vi "Set Resistance Colors.vi"(8 "error in (no error)":errorcluster, 11 "Data in":T1 {"#Bands" min=3 max=6 step=1}) -> (0 "error out":errorcluster, 3 "Data out":T1 {"#Bands" min=3 max=6 step=1})   [LabVIEW 2018]
uses:
  Data--cluster.ctl
  Digit--enum.ctl
  Multiplier--enum.ctl
  Tolerance--enum.ctl
  Temp Coeficient--enum.ctl
  E-Series Reader/Series Data--cluster.ctl
  In Low Series--cluster.ctl
  In Mid-High Series--cluster.ctl
  Number of Bands--number.ctl
  Enum to Color Converters/Enum to Color Converters.lvlib
  E-Series Reader/E-Series Reader.lvlib
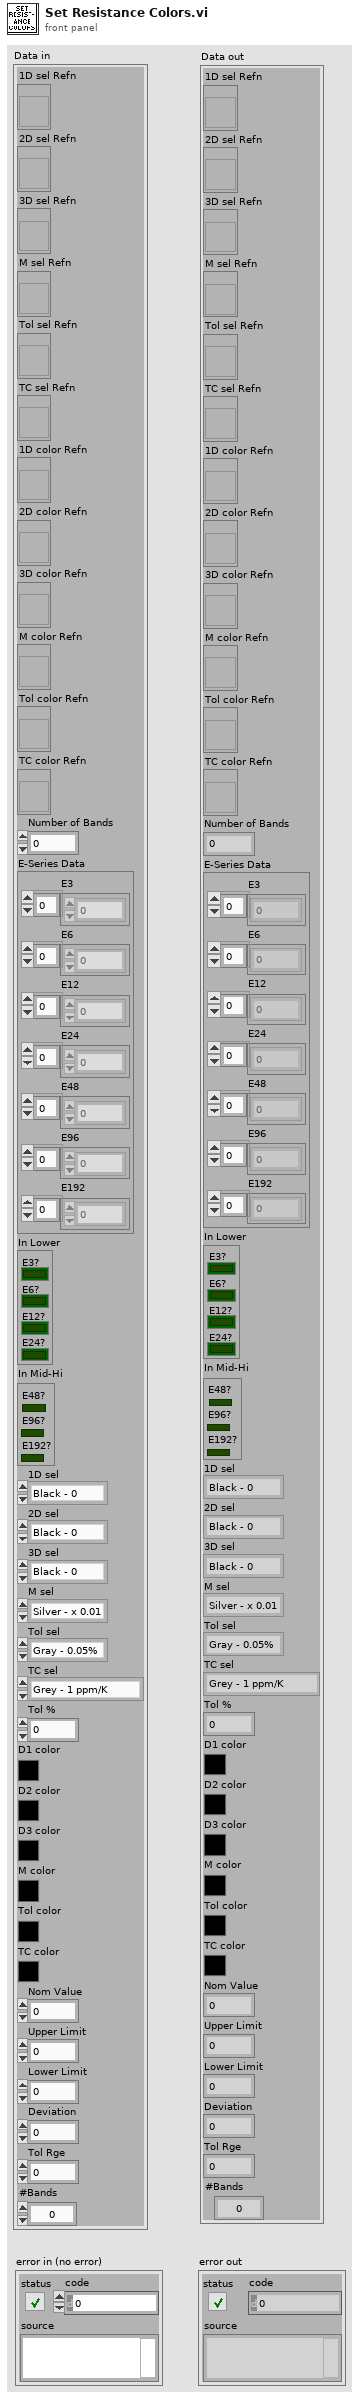
[diagram p1: front panel]
types:
  T1 = typedef "Data--cluster.ctl" = cluster{"1D sel Refn":refnum<vi>, "2D sel Refn":refnum<vi>, "3D sel Refn":refnum<vi>, "M sel Refn":refnum<vi>, "Tol sel Refn":refnum<vi>, "TC sel Refn":refnum<vi>, "1D color Refn":refnum<vi>, "2D color Refn":refnum<vi>, "3D color Refn":refnum<vi>, "M color Refn":refnum<vi>, "Tol color Refn":refnum<vi>, "TC color Refn":refnum<vi>, "Number of Bands":u8, "E-Series Data":T2, "In Lower":T3, "In Mid-Hi":T4, "1D sel":T5, "2D sel":T5, "3D sel":T5, "M sel":T6, "Tol sel":T7, "TC sel":T8, "Tol %":dbl, "D1 color":u32, "D2 color":u32, "D3 color":u32, "M color":u32, "Tol color":u32, "TC color":u32, "Nom Value":dbl, "Upper Limit":dbl, "Lower Limit":dbl, "Deviation":dbl, "Tol Rge":dbl, "#Bands":T9}
  T2 = typedef "E-Series Reader.lvlib/series data--cluster.ctl" = cluster{"E3":u16[], "E6":u16[], "E12":u16[], "E24":u16[], "E48":u16[], "E96":u16[], "E192":u16[]}
  T3 = typedef "In low series--cluster.ctl" = cluster{"E3?":bool, "E6?":bool, "E12?":bool, "E24?":bool}
  T4 = typedef "In mid-high series--cluster.ctl" = cluster{"E48?":bool, "E96?":bool, "E192?":bool}
  T5 = typedef "digit--enum.ctl" = enum16{"Black - 0", "Brown - 1", "Red - 2", "Orange - 3", "Yellow - 4", "Green - 5", "Blue - 6", "Violet - 7", "Grey - 8", "White - 9"}
  T6 = typedef "multiplier--enum.ctl" = enum16{"Silver - x 0.01", "Gold - x 0.1 ", "Black - x 1", "Brown - x 10", "Red - x 100", "Orange - x 1k", "Yellow - x 10k", "Green - 100k", "Blue - x 1M", "Violet - x10 M", "Grey - x 100M", "White - x 1G"}
  T7 = typedef "tolerance--enum.ctl" = enum16{"Gray - 0.05%", "Violet - 0.1%", "Blue - 0.25%", "Green - 0.5%", "Brown - 1%", "Red - 2%", "Gold - 5%", "Silver - 10%", "None - 20%"}
  T8 = typedef "temp coeficient--enum.ctl" = enum16{"Grey - 1 ppm/K", "Violet - 5 ppm/K", "Blue - 10 ppm/K", "Green - 20 ppm/K", "Yellow - 25 ppm/K", "Orange - 15 ppm/K", "Red - 50 ppm/K", "Brown - 100 ppm/K", "Black - 250 ppm/K"}
  T9 = typedef "Number of Bands--number.ctl" = u8
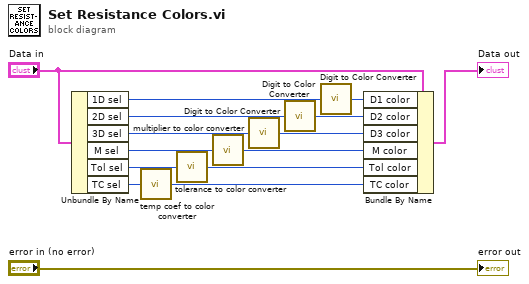
[diagram p0: block diagram]
diagram:
  n1 = Unbundle By Name("Data in") -> ("1D sel"=w2:T5, "2D sel"=w3:T5, "3D sel"=w12:T5, "M sel"=w8:T6, "Tol sel"=w9:T7, "TC sel"=w14:T8)
  n2 = call "temp coef to color converter.vi"("TC select"=w14) -> ("TC Color"=w15:u32)  [unwired: 6 in]
  n3 = call "tolerance to color converter.vi"("To select"=w9) -> ("Tol Color"=w10:u32)  [unwired: 6 in]
  n4 = call "multiplier to color converter.vi"("Mul select"=w8) -> ("Mult Color"=w11:u32)  [unwired: 6 in]
  n5 = call "Digit to Color Converter.vi"("D select"=w12) -> ("D Color"=w13:u32)  [unwired: 4 in]
  n6 = call "Digit to Color Converter.vi"("D select"=w3) -> ("D Color"=w7:u32)  [unwired: 4 in]
  n7 = call "Digit to Color Converter.vi"("D select"=w2) -> ("D Color"=w6:u32)  [unwired: 4 in]
  n8 = Bundle By Name(cluster="Data in", "D1 color"=w6, "D2 color"=w7, "D3 color"=w13, "M color"=w11, "Tol color"=w10, "TC color"=w15) -> (→"Data out":T1)
  "error out" <- "error in (no error)"
